vi "BallPresent.vi"(7 "Group":string, 9 "Present?":bool, 10 "SizeAndLocation":T1, 11 "Image in":T2) -> (3 "Image out":T2)   [LabVIEW 2015]
uses:
  <vilib>/vision/Image Controls.llb/IMAQ Image.ctl
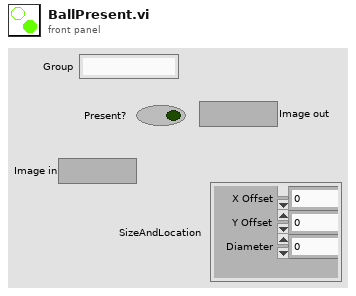
[diagram p1: front panel]
types:
  T1 = cluster{"X Offset":i32, "Y Offset":i32, "Diameter":i32}
  T2 = typedef "IMAQ Image.ctl" = refnum<image>
  T3 = cluster{"Left":i32, "Top":i32, "Right":i32, "Bottom":i32}
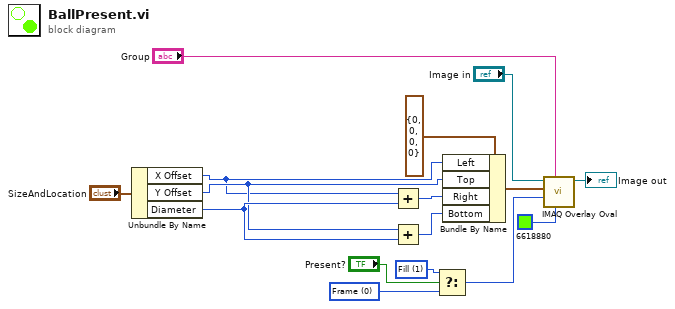
[diagram p0: block diagram]
diagram:
  w8 = u32 1 items=["Frame", "Fill"] ("Drawing Mode (Frame)")
  w10 = u32 0 items=["Frame", "Fill"] ("Drawing Mode (Frame)")
  n1 = Unbundle By Name("SizeAndLocation") -> ("X Offset"=w2:i32, "Y Offset"=w3:i32, "Diameter"=w4:i32)
  n2 = Add(x=w2, y=w4) -> (x+y=w15:i32)
  n3 = Add(x=w3, y=w4) -> (x+y=w14:i32)
  n4 = Select(t=w8, s="Present?", f=w10) -> (s? t:f=w9:u32)
  n5 = Bundle By Name(cluster=T3 {"Left"=0, "Top"=0, "Right"=0, "Bottom"=0} ("Bounding Rectangle"), "Left"=w2, "Top"=w3, "Right"=w15, "Bottom"=w14) -> (w13:T3)
  n6 = call "IMAQ Overlay Oval"("Color"=u32 6618880, "Group"="Group", "Drawing Mode (Frame)"=w9, "Bounding Rectangle"=w13, "Image"="Image in") -> ("Image Out"=→"Image out":T2)  [unwired: 5 in, 1 out]
